vi "Testbench.vi"() -> ()   [LabVIEW 2012]
uses:
  <instrlib>/Stanford Research SR865/Stanford Research SR865.lvlib
panel:
  in  "Chopper Frequency":dbl(knob) scale=100.0..1000.0
  in  "Chopper Phase":dbl(knob) scale=0.0..180.0
  in  "Numeric":i32
  in  "Run VI":bool=TRUE
  out "String":string
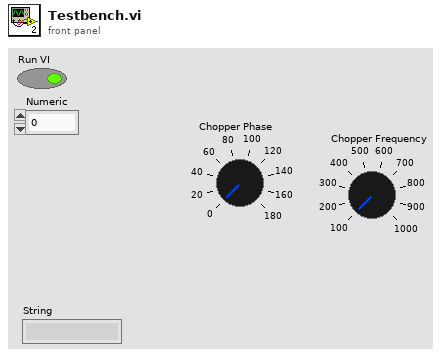
[diagram p1: front panel]
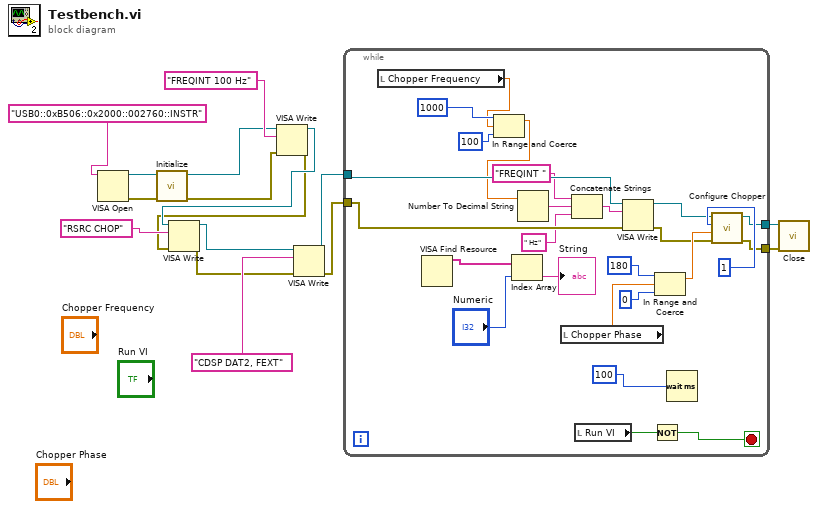
[diagram p0: block diagram]
diagram:
  n1 = VISA Open(VISA resource name="USB0::0xB506::0x2000::002760::INSTR") -> (VISA resource name=w15:refnum<visa-resource-name>, error out=w14:errorcluster)  [unwired: 4 in]
  n2 = call <instrlib>:"Initialize.vi"("error in (no error)"=w14, "VISA resource name"=w15) -> ("error out"=w1:errorcluster, "VISA resource name out"=w6:refnum<visa-resource-name>)  [unwired: 8 in]
  n3 = VISA Write(VISA resource name=w6, write buffer="FREQINT 100 Hz", error in (no error)=w1) -> (VISA resource name out=w5:refnum<visa-resource-name>, error out=w2:errorcluster)  [unwired: 1 out]
  n4 = VISA Write(VISA resource name=w5, write buffer="RSRC CHOP", error in (no error)=w2) -> (VISA resource name out=w4:refnum<visa-resource-name>, error out=w3:errorcluster)  [unwired: 1 out]
  n5 = VISA Write(VISA resource name=w4, write buffer="CDSP DAT2, FEXT", error in (no error)=w3) -> (VISA resource name out=w8:refnum<visa-resource-name>, error out=w9:errorcluster)  [unwired: 1 out]
  n6 = while {
    tunnel: w8 -> [w30]
    tunnel: w9 -> [w29]
    tunnel: [w28] -> w13
    tunnel: [w27] -> w12
    stop <- w38 stop-if-true
    n7 = local read "Chopper Frequency"() -> (w24:dbl)
    n8 = VISA Find Resource() -> (3:w40:string[])  [unwired: 3 in, 2 out]
    n9 = In Range and Coerce(upper limit=1000, x=w24, lower limit=100) -> (coerced(x)=w20:dbl)  [unwired: 1 out]
    n10 = Index Array(array=w40, index="Numeric") -> (element=→"String":string)
    n11 = Number To Decimal String(number=w20) -> (decimal integer string=w22:string)  [unwired: 1 in]
    n12 = local read "Chopper Phase"() -> (w31:dbl)
    n13 = Concatenate Strings("FREQINT ", w22, " Hz") -> (w19:string)
    n14 = local read "Run VI"() -> (w37:bool)
    n15 = VISA Write(VISA resource name=w30, write buffer=w19, error in (no error)=w29) -> (VISA resource name out=w17:refnum<visa-resource-name>, error out=w18:errorcluster)  [unwired: 1 out]
    n16 = Not(x=w37) -> (.not. x?=w38:bool)
    n17 = In Range and Coerce(upper limit=180, x=w31, lower limit=0) -> (coerced(x)=w33:dbl)  [unwired: 1 out]
    n18 = Wait (ms)(milliseconds to wait=100) -> ()  [unwired: 1 out]
    n19 = call <instrlib>:"Configure Chopper.vi"("error in (no error)"=w18, "Blade Phase (0 Degree)"=w33, "Chopper Blade (0: 6-slot)"=1, "VISA resource name"=w17) -> ("error out"=w27:errorcluster, "VISA resource name out"=w28:refnum<visa-resource-name>)  [unwired: 6 in]
  }
  n20 = call <instrlib>:"Close.vi"("error in (no error)"=w12, "VISA resource name"=w13) -> ()  [unwired: 9 in, 1 out]
